vi "Tegam4040 -- Test Set-GetInputImpedance.vi"() -> ()   [LabVIEW 2010]
panel:
  out "error out":errorcluster
  out "Get Input Impedance":enum16{" 1 MOhm", "50 Ohm"}(ring)
  in  "Set Input Impedance":enum16{" 1 MOhm", "50 Ohm"}(ring)
  in  "Tegam4040 Resource":refnum<visa-resource-name>
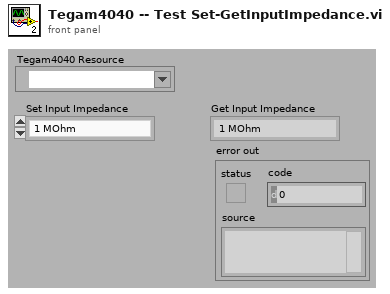
[diagram p1: front panel]
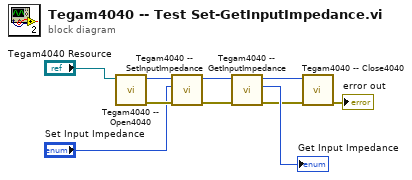
[diagram p0: block diagram]
diagram:
  n1 = call "Tegam4040 -- Open4040.vi"("VISA Resource In"="Tegam4040 Resource") -> ("error out"=w8:errorcluster, "Instrument Session Handle"=w9:u32)  [unwired: 9 in]
  n2 = call "Tegam4040 -- SetInputImpedance.vi"("error in (no error)"=w8, "Input Impedance"="Set Input Impedance", "Instrument Session Handle In"=w9) -> ("error out"=w7:errorcluster, "Instrument Session Handle Out (dupl)"=w6:u32)  [unwired: 7 in]
  n3 = call "Tegam4040 -- GetInputImpedance.vi"("error in (no error)"=w7, "Instrument Session Handle In"=w6) -> ("error out"=w3:errorcluster, "Input Impedance"=→"Get Input Impedance":enum16{" 1 MOhm", "50 Ohm"}, "Instrument Session Handle Out (dupl)"=w2:u32)  [unwired: 7 in]
  n4 = call "Tegam4040 -- Close4040.vi"("error in (no error)"=w3, "Instrument Session Handle"=w2) -> ("error out"=→"error out":errorcluster)  [unwired: 9 in]
